vi "FGV_button.vi"(10 "Reset":bool, 11 "Set":bool) -> (3 "out":bool)   [LabVIEW 2022 SP3]
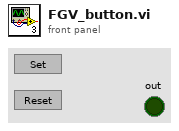
[diagram p1: front panel]
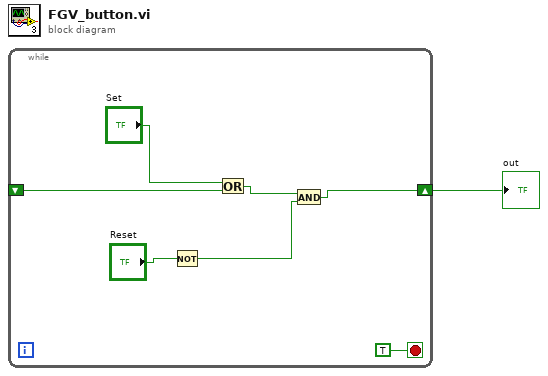
[diagram p0: block diagram]
diagram:
  n1 = while {
    shift-right: [w3] -> w1
    shift-left: _ -> [w2]
    stop <- TRUE stop-if-true
    n2 = Not(x="Reset") -> (.not. x?=w4:bool)
    n3 = Or(x="Set", y=w2) -> (x .or. y?=w6:bool)
    n4 = And(x=w6, y=w4) -> (x .and. y?=w3:bool)
  }
  "out" <- w1
